vi "Speed of VIight FPGA_v4.vi"() -> ()   [LabVIEW 2026]
uses:
  <vilib>/rvi/Emulation/niFpgaGetClockAttributes.vi
  <vilib>/rvi/Emulation/niFpgaSctlEmulationGetInTimedLoop.vi
  <vilib>/rvi/Emulation/niFpgaEmulationReportErrorSimple.vi
  <instrlib>/_niInstr/Basic Elements/v1/FPGA/Private/Count Up U16.vi
  <vilib>/rvi/eio/common/nirviEmuTemplateMethod_errors.vi
  <vilib>/rvi/Emulation/niFpgaCriticalErrorInLSC.vi
  <vilib>/rvi/Emulation/niFpgaProcessEmulError.vi
  <vilib>/eio/EIONode/EIONode.xnode
  <instrlib>/_niInstr/Basic Elements/v1/FPGA/niInstr Basic Elements v1 FPGA.lvlib
panel:
  out "Play Sound 2":bool
  in  "Frequency Array":fxp<+,32,0>[](array[numeric])=[1.100008375942707e-05, 1.165410503745079e-05, 1.3081356883049011e-05, 1.3859011232852936e-05, 1.7461366951465607e-05, 1.8499791622161865e-05, 2.1999934688210487e-05, 2.330821007490158e-05, 2.6162713766098022e-05, 2.7718255296349525e-05]
  in  "Tone 1 Length":u32=15000
  out "Bonus On?":bool
  in  "Tone Length":u32=40000
  in  "Audio Loop Stop":bool
  in  "reset":bool
  out "sine out":i16
  in  "Count(uSec)":u32=10
  out "Play Sound":bool
  out "Idle Loop":i32
  in  "Period":u16=100
  in  "Idle Pattern":u16[](array[numeric])=[0, 0, 0, 0, 0, 0, 0, 0, 0, 0, 0, 0, 0, 0, 0, 0, 0, 0, 0, 0, 0, 0, 0, 0, 0, 0, 0, 0, 0, 0, 0, 0, 0, 0, 0, 0, 0, 0, 0, 0, 0, 0, 0, 0, 0]
  out "Main Loop Complete":bool
  out "Player 2 Output 5":bool[](array[boolean])
  out "Player 1 Output 5":bool[](array[boolean])
  out "Initial 6 Random Numbers":u8[](array[numeric])
  out "Player 2 Bonus":u8
  out "Player 1 Bonus":u8
  in  "Max Bonus":u8=5
  in  "Bonus Threshold":u64=3000
  out "Intial Random Arrays":u8[](array[numeric])
  out "Player2 Input":bool[](array[boolean])
  out "Player1 Input":bool[](array[boolean])
  out "Player 2 Output 4":bool[](array[boolean])
  out "Player 2 Output 3":bool[](array[boolean])
  out "Player 2 Output 2":bool[](array[boolean])
  out "Player 2 Output 1":bool[](array[boolean])
  out "Player 1 Output 4":bool[](array[boolean])
  out "Player 1 Output 3":bool[](array[boolean])
  out "Player 1 Output 2":bool[](array[boolean])
  out "Player 2 Score":u32
  out "Player 2 Timer":u64
  out "Player 1 Score":u32
  out "Player 1 Timer":u64
  out "Main Loop":i32
  out "Closing Loop":i32
  out "Element to change 2":i32
  out "Element to change":i32
  out "Measured Main Loop Ticks":u32
  in  "Main Loop Timer":u32=1 caption="Main Loop Timer (uSec)"
  out "Player2 Output Number":u32
  out "Player1 Output Number":u32
  out "Initialized Array 2":bool[](array[boolean])
  out "Initialized Array 1":bool[](array[boolean])
  out "Random Number":u8
  in  "Random Number Max":u8=20
  out "Current State":i16
  out "Blue2":bool
  out "Green3":bool
  out "Green2":bool
  out "Blue1":bool
  out "Green1":bool
  out "Player 1 Output":bool[](array[boolean])
  in  "Game Length (s)":u32=45
  in  "Stop Closing Loop":bool
  in  "Stop Main Loop":bool
  in  "Stop Idle":bool
  in  "Global Stop":bool
  # "100kHz"
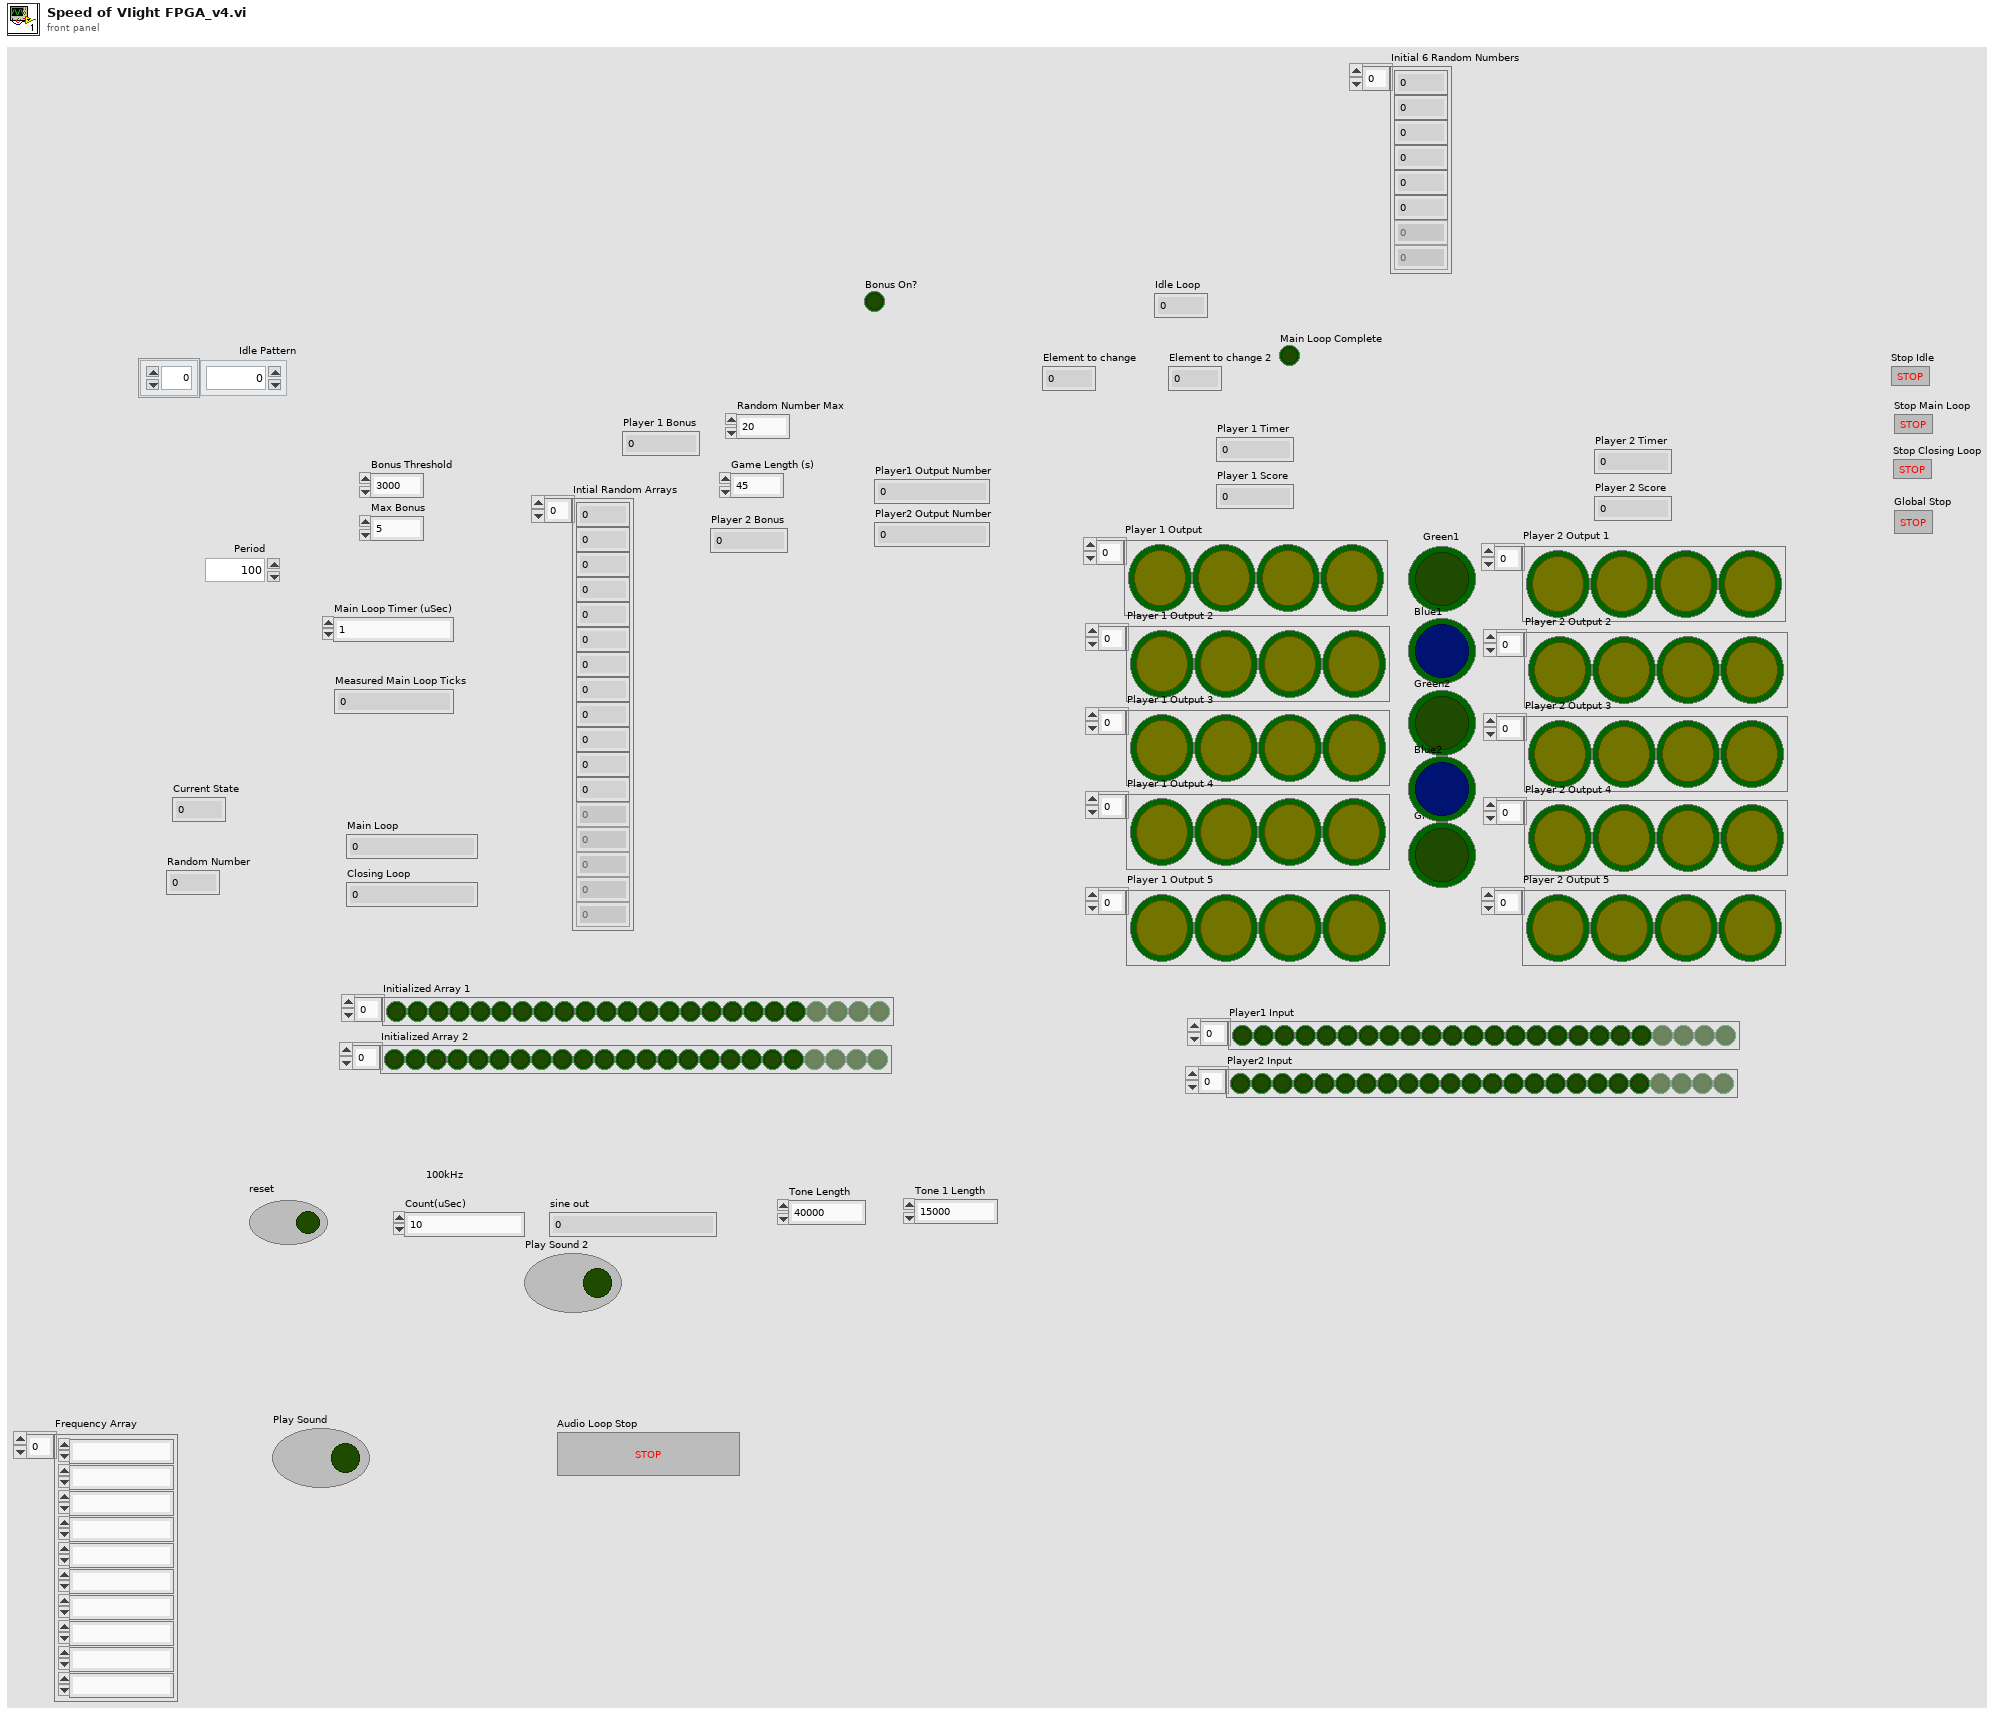
[diagram p1: front panel]
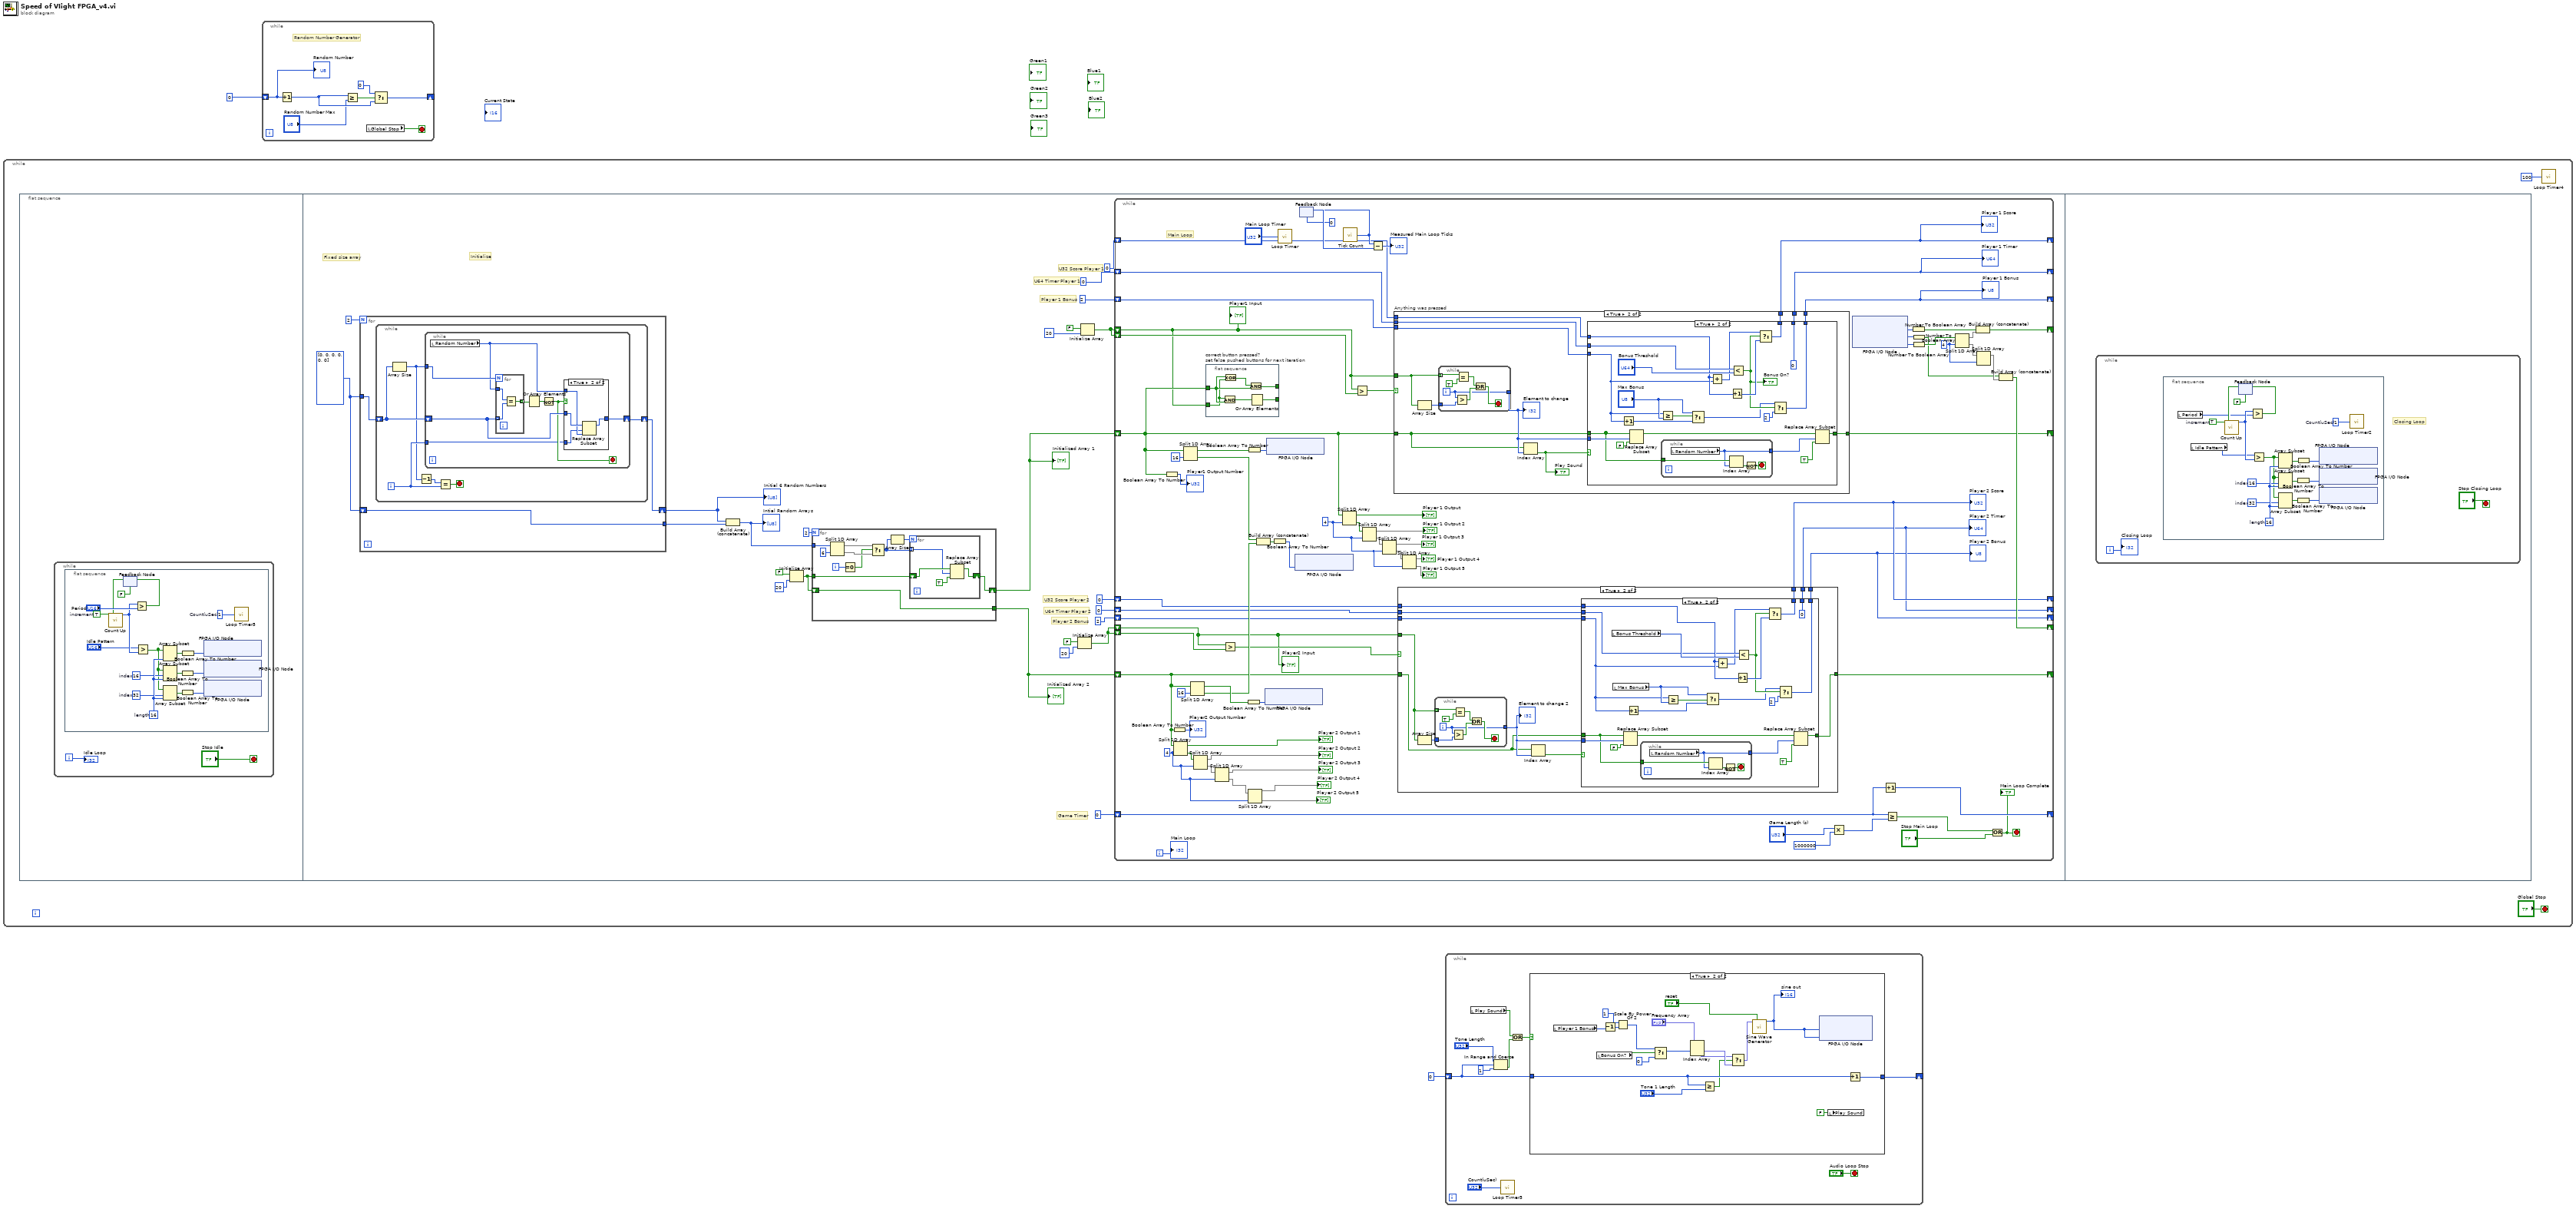
[diagram p0: block diagram]
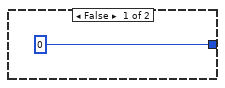
[diagram p2: hidden frame]
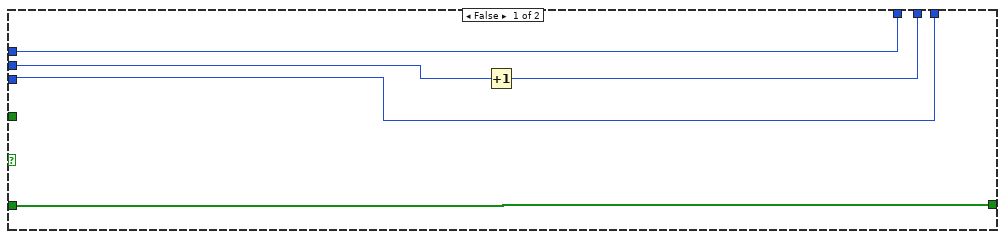
[diagram p4: hidden frame]
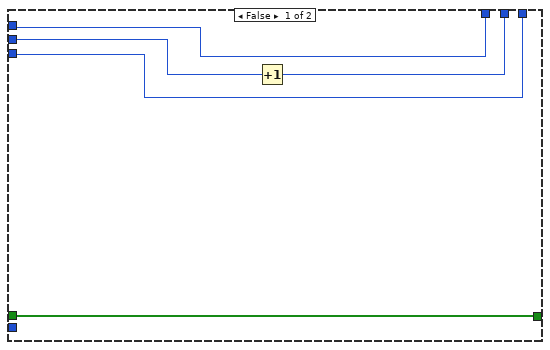
[diagram p5: hidden frame]
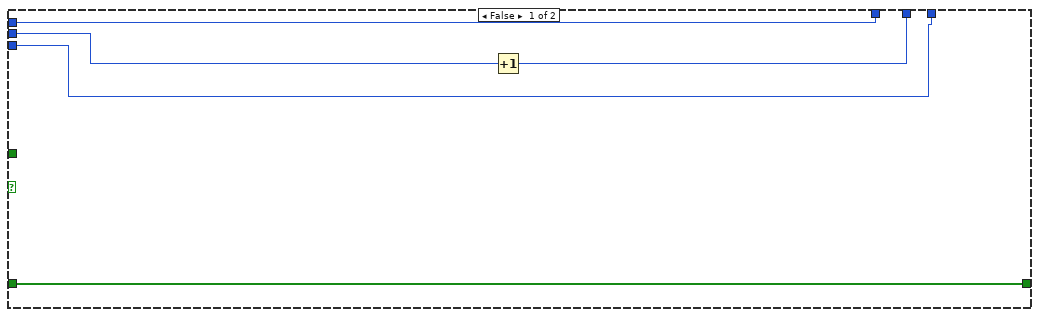
[diagram p6: hidden frame]
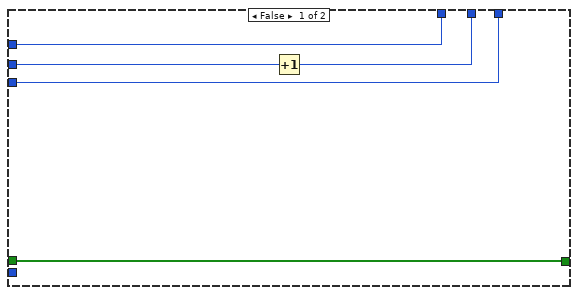
[diagram p7: hidden frame]
diagram:
  n1 = while {
    stop <- "Global Stop" stop-if-true
    n2 = flat-sequence {
      frame #0 {
        n3 = while {
          i -> [w5]
          stop <- "Stop Idle" stop-if-true
          n4 = flat-sequence {
            frame #0 {
              w11 = 32  # index
              w12 = 16  # index
              w13 = 16  # length
              w20 = u16 1  # Count(uSec)
              w23 = TRUE  # increment
              n5 = feedback #1(FALSE) -> (w19:bool)
              n6 = call-poly <instrlib>:"Count Up.vi"("increment"=w23, "reset"=w19) -> ("count out"=w18:u16)  [unwired: 13 in]
              n7 = Greater?(x=w18, y="Period") -> (0:w21:bool)
              n8 = feedback-in #1(w21) -> ()
              n9 = Greater?(x="Idle Pattern", y=w18) -> (0:w9:bool[])
              n10 = Array Subset(array=w9, length=w13) -> (w7:bool[])  [unwired: 1 in]
              n11 = Array Subset(array=w9, index=w12, length=w13) -> (w8:bool[])
              n12 = Array Subset(array=w9, index=w11, length=w13) -> (w10:bool[])
              n13 = Boolean Array To Number(Boolean array=w8) -> (number=w15:u16)
              n14 = Boolean Array To Number(Boolean array=w10) -> (number=w14:u16)
              n15 = Boolean Array To Number(Boolean array=w7) -> (number=w16:u16)
              n16 = xnode "FPGA I/O Node"("Bank-01/DO15:0"=w16) -> ()  [unwired: 1 in, 1 out]
              n17 = xnode "FPGA I/O Node"("Bank-02/DO15:0"=w15) -> ()  [unwired: 1 in, 1 out]
              n18 = xnode "FPGA I/O Node"("Bank-03/DO15:0"=w14) -> ()  [unwired: 1 in, 1 out]
              n19 = call "Loop Timer5"("Count(uSec)"=w20) -> ()  [unwired: 1 out]
            }
          }
          "Idle Loop" <- w5
        }
      }
      frame #1 {
        w30 = u8[] [0, 0, 0, 0, 0, 0] ("Initial Random Numbers")
        # "Player 2 Bonus"
        # "Player 1 Bonus"
        # "Initialize"
        # "Fixed size array"
        # "Game Timer"
        # "U32 Score Player 2"
        # "U32 Score Player 1"
        # "U64 Timer Player 2"
        # "U64 Timer Player 1"
        n20 = for {
          N: 2 -> [_]
          tunnel: w30 -> [w66]
          shift-right: [w65] -> w29
          shift-left: w30 -> [w64]
          tunnel: [w64] -> w28
          n21 = while {
            shift-right: [w69] -> w65
            shift-left: w66 -> [w70]
            i -> [w72]
            stop <- w71 stop-if-true
            n22 = Array Size(array=w70) -> (size(s)=w67:i32)
            n23 = Decrement(x=w67) -> (x-1=w68:i32)
            n24 = while {
              tunnel: w72 -> [w74]
              shift-right: [w75] -> w69
              shift-left: w70 -> [w77]
              tunnel: w67 -> [w80]
              stop <- w76 stop-if-true
              n25 = local read "Random Number"() -> (w73:u8)
              n26 = for {
                N: w80 -> [_]
                tunnel: w77 -> [w87] mode=indexing
                tunnel: w73 -> [w88]
                tunnel: [w86] -> w79 mode=indexing
                n27 = Equal?(x=w88, y=w87) -> (x = y?=w86:bool)
              }
              n28 = Or Array Elements(Boolean array=w79) -> (logical OR=w78:bool)
              n29 = Not(x=w78) -> (.not. x?=w76:bool)
              n30 = case shown="True" w76 {
                tunnel: w77 -> [w81 w85]
                tunnel: [w81 w84] -> w75
                tunnel: w73 -> [_ w83]
                tunnel: w74 -> [_ w82]
                frame False {
                }
                frame True {
                  n31 = Replace Array Subset(array=w85, new element=w83, index=w82) -> (w84:u8[])
                }
              }
            }
            n32 = Equal?(x=w68, y=w72) -> (x = y?=w71:bool)
          }
        }
        "Initial 6 Random Numbers" <- w29
        n33 = Build Array (concatenate)(w29, w28) -> (w27:u8[])
        "Intial Random Arrays" <- w27
        n34 = Initialize Array(FALSE ("Boolean"), 20 ("dimension size")) -> (w31:bool[])
        n35 = for {
          N: 2 -> [_]
          tunnel: w31 -> [w58]
          tunnel: w27 -> [w56]
          shift-right: [w59] -> w26
          shift-left: w31 -> [w49]
          tunnel: [w49] -> w25
          i -> [w52]
          n36 = Split 1D Array(array=w56, index=6) -> (first subarray=w53:u8[], second subarray=w54:u8[])
          n37 = Equal To 0?(x=w52) -> (x = 0?=w51:bool)
          n38 = Select(t=w53, s=w51, f=w54) -> (s? t:f=w50:u8[])
          n39 = Array Size(array=w50) -> (size(s)=w57:i32)
          n40 = for {
            N: w57 -> [_]
            tunnel: w50 -> [w60] mode=indexing
            shift-right: [w63] -> w59
            shift-left: w58 -> [w62]
            n41 = Replace Array Subset(array=w62, new element=TRUE ("new element/subarray"), index=w60) -> (w63:bool[])
          }
        }
        "Initialized Array 1" <- w26
        "Initialized Array 2" <- w25
        n42 = Initialize Array(FALSE ("Boolean"), 20 ("dimension size")) -> (w32:bool[])
        n43 = Initialize Array(FALSE ("Boolean"), 20 ("dimension size")) -> (w35:bool[])
        n44 = while {
          shift-right: [w110] -> _
          shift-left: u64 0 -> [w113]
          shift-right: [w104] -> _
          shift-left: u64 0 -> [w108]
          shift-right: [w111] -> _
          shift-left: u32 0 -> [w112]
          shift-right: [w105] -> _
          shift-left: u32 0 -> [w106]
          shift-right: [w164] -> _
          shift-left: u32 0 -> [w165]
          shift-right: [w134] -> _
          shift-left: w26 -> [w91]
          shift-right: [w131] -> _
          shift-left: w25 -> [w125]
          shift-right: [w139] -> _
          shift-left: w35 -> [w89]
          shift-right: [w138] -> _
          shift-left: w32 -> [w114]
          shift-left: w35 -> [w137]
          shift-left: w32 -> [w133]
          shift-right: [w109] -> _
          shift-left: u8 2 -> [w90]
          shift-right: [w103] -> _
          shift-left: u8 2 -> [w107]
          i -> [w127]
          stop <- w92 stop-if-true
          w93 = 4 ("index")
          w100 = 4 ("index")
          w145 = 4 ("index")
          # "Main Loop"
          n45 = Boolean Array To Number(Boolean array=w91) -> (number=→"Player1 Output Number":u32)
          n46 = Boolean Array To Number(Boolean array=w125) -> (number=→"Player2 Output Number":u32)
          n47 = Split 1D Array(array=w125, index=w100) -> (first subarray=→"Player 2 Output 1":bool[], second subarray=w123:bool[])
          n48 = Split 1D Array(array=w91, index=16) -> (first subarray=w135:bool[], second subarray=w155:bool[])
          n49 = Split 1D Array(array=w125, index=16) -> (first subarray=w158:bool[], second subarray=w154:bool[])
          n50 = Split 1D Array(array=w123, index=w100) -> (first subarray=→"Player 2 Output 2":bool[], second subarray=w121:bool[])
          n51 = flat-sequence "correct button pressed?\nset false pushed buttons for next iteration" {
            tunnel: [w171] -> _
            tunnel: w91 -> [w169]
            tunnel: w89 -> [w168]
            tunnel: [w167] -> _
            frame #0 {
              n52 = And(x=w168, y=w169) -> (x .and. y?=w170:bool[])
              n53 = Exclusive Or(1:w168, 2:w169) -> (0:w172:bool[])
              n54 = And(x=w172, y=w169) -> (x .and. y?=w171:bool[])
              n55 = Or Array Elements(Boolean array=w170) -> (logical OR=w167:bool)
            }
          }
          n56 = Split 1D Array(array=w121, index=w100) -> (first subarray=→"Player 2 Output 3":bool[], second subarray=w98:bool[])
          n57 = Greater?(x=w114, y=w133) -> (0:w132:bool)
          n58 = Boolean Array To Number(Boolean array=w158) -> (number=w157:u32)
          n59 = Boolean Array To Number(Boolean array=w135) -> (number=w160:u32)
          n60 = Split 1D Array(array=w98, index=w100) -> (first subarray=→"Player 2 Output 4":bool[], second subarray=→"Player 2 Output 5":bool[])
          n61 = Build Array (concatenate)(w155, w154) -> (w153:bool[])
          n62 = xnode "FPGA I/O Node"("Bank-02/DO15:0"=w157) -> ()  [unwired: 1 in, 1 out]
          n63 = xnode "FPGA I/O Node"("Bank-01/DO15:0"=w160) -> ()  [unwired: 1 in, 1 out]
          n64 = Boolean Array To Number(Boolean array=w153) -> (number=w152:u32)
          n65 = call "Loop Timer"("Count(uSec)"="Main Loop Timer") -> ()  [unwired: 1 out]
          n66 = xnode "FPGA I/O Node"("Bank-03/DO15:0"=w152) -> ()  [unwired: 1 in, 1 out]
          n67 = feedback #2(u32 0) -> (w142:u32)
          n68 = Split 1D Array(array=w91, index=w93) -> (first subarray=→"Player 1 Output":bool[], second subarray=w119:bool[])
          n69 = call "Tick Count"() -> ("Tick Count(Ticks)"=w141:u32)
          n70 = feedback-in #2(w141) -> ()
          n71 = Greater?(x=w89, y=w137) -> (0:w136:bool)
          n72 = Split 1D Array(array=w119, index=w93) -> (first subarray=→"Player 1 Output 2":bool[], second subarray=w118:bool[])
          n73 = Subtract(x=w141, y=w142) -> (x-y=→"Measured Main Loop Ticks":u32)
          n74 = Split 1D Array(array=w118, index=w93) -> (first subarray=→"Player 1 Output 3":bool[], second subarray=w96:bool[])
          n75 = case "Anything was pressed" shown="True" w136 {
            tunnel: [w232 w244] -> w134
            tunnel: w89 -> [_ w242]
            tunnel: w91 -> [w232 w240]
            tunnel: w113 -> [w230 w236]
            tunnel: [w229 w238] -> w110
            tunnel: w112 -> [w231 w237]
            tunnel: [w231 w239] -> w111
            tunnel: w90 -> [w228 w235]
            tunnel: [w228 w234] -> w109
            frame False {
              n76 = Increment(x=w230) -> (x+1=w229:u64)
            }
            frame True {
              n77 = Array Size(array=w242) -> (size(s)=w241:i32)
              n78 = while {
                tunnel: w242 -> [w282] mode=indexing
                tunnel: w241 -> [w278]
                tunnel: [w276] -> w243
                i -> [w276]
                stop <- w279 stop-if-true
                n79 = Greater?(x=w276, y=w278) -> (0:w277:bool)
                n80 = Equal?(x=w282, y=TRUE ("element")) -> (x = y?=w280:bool)
                n81 = Or(x=w280, y=w277) -> (x .or. y?=w279:bool)
              }
              "Element to change" <- w243
              n82 = Index Array(array=w240, index=w243) -> (element=w233:bool)
              "Play Sound" <- w233
              n83 = case shown="True" w233 {
                tunnel: w243 -> [_ w271]
                tunnel: [w249 w267] -> w244
                tunnel: w240 -> [w249 w265]
                tunnel: w237 -> [w248 w252]
                tunnel: w236 -> [w247 w263]
                tunnel: [w248 w261] -> w239
                tunnel: [w246 u64 0] -> w238
                tunnel: w235 -> [w245 w251]
                tunnel: [w245 w258] -> w234
                frame False {
                  n84 = Increment(x=w247) -> (x+1=w246:u64)
                }
                frame True {
                  n85 = Increment(x=w251) -> (x+1=w254:u8)
                  n86 = Replace Array Subset(array=w265, new element=FALSE ("new element/subarray"), index=w271) -> (w269:bool[])
                  n87 = Greater Or Equal?(x=w251, y="Max Bonus") -> (x >= y?=w256:bool)
                  n88 = while {
                    tunnel: [w272] -> w266
                    tunnel: w265 -> [w275]
                    stop <- w273 stop-if-true
                    n89 = local read "Random Number"() -> (w272:u8)
                    n90 = Index Array(array=w275, index=w272) -> (element=w274:bool)
                    n91 = Not(x=w274) -> (.not. x?=w273:bool)
                  }
                  n92 = Select(t="Max Bonus", s=w256, f=w254) -> (s? t:f=w253:u8)
                  n93 = Add(x=w252, y=w251) -> (x+y=w250:u32)
                  n94 = Increment(x=w252) -> (x+1=w262:u32)
                  n95 = Less?(x=w263, y="Bonus Threshold") -> (x < y?=w260:bool)
                  "Bonus On?" <- w260
                  n96 = Select(t=w250, s=w260, f=w262) -> (s? t:f=w261:u32)
                  n97 = Select(t=w253, s=w260, f=u8 2) -> (s? t:f=w258:u8)
                  n98 = Replace Array Subset(array=w269, new element=TRUE ("new element/subarray"), index=w266) -> (w267:bool[])
                }
              }
            }
          }
          "Player 1 Timer" <- w110
          "Player 1 Score" <- w111
          "Player 1 Bonus" <- w109
          n99 = case shown="True" w132 {
            tunnel: [w177 w185] -> w131
            tunnel: w114 -> [_ w187]
            tunnel: w125 -> [w177 w184]
            tunnel: w108 -> [w175 w182]
            tunnel: w107 -> [w173 w181]
            tunnel: w106 -> [w176 w183]
            tunnel: [w176 w179] -> w105
            tunnel: [w174 w180] -> w104
            tunnel: [w173 w178] -> w103
            frame False {
              n100 = Increment(x=w175) -> (x+1=w174:u64)
            }
            frame True {
              n101 = Array Size(array=w187) -> (size(s)=w186:i32)
              n102 = while {
                tunnel: w187 -> [w227] mode=indexing
                tunnel: w186 -> [w223]
                tunnel: [w221] -> w189
                i -> [w221]
                stop <- w224 stop-if-true
                n103 = Greater?(x=w221, y=w223) -> (0:w222:bool)
                n104 = Equal?(x=w227, y=TRUE ("element")) -> (x = y?=w225:bool)
                n105 = Or(x=w225, y=w222) -> (x .or. y?=w224:bool)
              }
              "Element to change 2" <- w189
              n106 = Index Array(array=w184, index=w189) -> (element=w188:bool)
              n107 = case shown="True" w188 {
                tunnel: w189 -> [_ w216]
                tunnel: [w194 w212] -> w185
                tunnel: w184 -> [w194 w210]
                tunnel: w183 -> [w190 w202]
                tunnel: w182 -> [w193 w197]
                tunnel: w181 -> [w191 w195]
                tunnel: [w192 u64 0] -> w180
                tunnel: [w191 w200] -> w178
                tunnel: [w190 w199] -> w179
                frame False {
                  n108 = Increment(x=w193) -> (x+1=w192:u64)
                }
                frame True {
                  n109 = local read "Bonus Threshold"() -> (w204:u64)
                  n110 = local read "Max Bonus"() -> (w203:u8)
                  n111 = Replace Array Subset(array=w210, new element=FALSE ("new element/subarray"), index=w216) -> (w214:bool[])
                  n112 = Increment(x=w195) -> (x+1=w198:u8)
                  n113 = while {
                    tunnel: [w217] -> w211
                    tunnel: w210 -> [w220]
                    stop <- w218 stop-if-true
                    n114 = local read "Random Number"() -> (w217:u8)
                    n115 = Index Array(array=w220, index=w217) -> (element=w219:bool)
                    n116 = Not(x=w219) -> (.not. x?=w218:bool)
                  }
                  n117 = Greater Or Equal?(x=w195, y=w203) -> (x >= y?=w206:bool)
                  n118 = Select(t=w203, s=w206, f=w198) -> (s? t:f=w205:u8)
                  n119 = Add(x=w202, y=w195) -> (x+y=w196:u32)
                  n120 = Increment(x=w202) -> (x+1=w209:u32)
                  n121 = Less?(x=w197, y=w204) -> (x < y?=w208:bool)
                  n122 = Select(t=w196, s=w208, f=w209) -> (s? t:f=w199:u32)
                  n123 = Select(t=w205, s=w208, f=u8 2) -> (s? t:f=w200:u8)
                  n124 = Replace Array Subset(array=w214, new element=TRUE ("new element/subarray"), index=w211) -> (w212:bool[])
                }
              }
            }
          }
          "Player 2 Timer" <- w104
          "Player 2 Score" <- w105
          "Player 2 Bonus" <- w103
          n125 = Split 1D Array(array=w96, index=w93) -> (first subarray=→"Player 1 Output 4":bool[], second subarray=→"Player 1 Output 5":bool[])
          n126 = Multiply(x="Game Length (s)", y=u32 1000000) -> (x*y=w128:u32)
          n127 = xnode "FPGA I/O Node"() -> ("Bank-01/DI15:0"=w151:u16, "Bank-02/DI15:0"=w150:u16, "Bank-03/DI15:0"=w149:u16)  [unwired: 3 in, 3 out]
          n128 = Increment(x=w165) -> (x+1=w164:u32)
          n129 = Greater Or Equal?(x=w165, y=w128) -> (x >= y?=w163:bool)
          n130 = Number To Boolean Array(number=w151) -> (Boolean array=w147:bool[])
          n131 = Number To Boolean Array(number=w150) -> (Boolean array=w101:bool[])
          n132 = Number To Boolean Array(number=w149) -> (Boolean array=w102:bool[])
          n133 = Split 1D Array(array=w102, index=w145) -> (first subarray=w146:bool[], second subarray=w144:bool[])
          n134 = Build Array (concatenate)(w147, w146) -> (w139:bool[])
          n135 = Split 1D Array(array=w144, index=w145) -> (first subarray=w143:bool[])  [unwired: 1 out]
          n136 = Or(x=w163, y="Stop Main Loop") -> (x .or. y?=w92:bool)
          "Main Loop Complete" <- w92
          n137 = Build Array (concatenate)(w101, w143) -> (w138:bool[])
          "Main Loop" <- w127
          "Player1 Input" <- w89
          "Player2 Input" <- w114
        }
      }
      frame #2 {
        n138 = while {
          i -> [w283]
          stop <- "Stop Closing Loop" stop-if-true
          # "Closing Loop"
          n139 = flat-sequence {
            frame #0 {
              w291 = 32  # index
              w292 = 16  # index
              w293 = 16  # length
              w299 = u16 1  # Count(uSec)
              w302 = TRUE  # increment
              n140 = local read "Period"() -> (w285:u16)
              n141 = local read "Idle Pattern"() -> (w286:u16[])
              n142 = feedback #3(FALSE) -> (w298:bool)
              n143 = call-poly <instrlib>:"Count Up.vi"("increment"=w302, "reset"=w298) -> ("count out"=w297:u16)  [unwired: 13 in]
              n144 = Greater?(x=w297, y=w285) -> (0:w300:bool)
              n145 = feedback-in #3(w300) -> ()
              n146 = Greater?(x=w286, y=w297) -> (0:w289:bool[])
              n147 = Array Subset(array=w289, length=w293) -> (w287:bool[])  [unwired: 1 in]
              n148 = Array Subset(array=w289, index=w292, length=w293) -> (w288:bool[])
              n149 = Array Subset(array=w289, index=w291, length=w293) -> (w290:bool[])
              n150 = Boolean Array To Number(Boolean array=w288) -> (number=w295:u16)
              n151 = Boolean Array To Number(Boolean array=w290) -> (number=w294:u16)
              n152 = Boolean Array To Number(Boolean array=w287) -> (number=w296:u16)
              n153 = xnode "FPGA I/O Node"("Bank-01/DO15:0"=w296) -> ()  [unwired: 1 in, 1 out]
              n154 = xnode "FPGA I/O Node"("Bank-02/DO15:0"=w295) -> ()  [unwired: 1 in, 1 out]
              n155 = xnode "FPGA I/O Node"("Bank-03/DO15:0"=w294) -> ()  [unwired: 1 in, 1 out]
              n156 = call "Loop Timer2"("Count(uSec)"=w299) -> ()  [unwired: 1 out]
            }
          }
          "Closing Loop" <- w283
        }
      }
    }
    n157 = call "Loop Timer4"("Count(mSec)"=u32 100 ("millisecond multiple")) -> ()  [unwired: 1 out]
  }
  n158 = while {
    shift-right: [w307] -> _
    shift-left: u8 0 -> [w309]
    stop <- w303 stop-if-true
    # "Random Number Generator"
    n159 = Increment(x=w309) -> (x+1=w306:u8)
    n160 = Greater Or Equal?(x=w306, y="Random Number Max") -> (x >= y?=w305:bool)
    n161 = local read "Global Stop"() -> (w303:bool)
    n162 = Select(t=u8 0, s=w305, f=w306) -> (s? t:f=w307:u8)
    "Random Number" <- w309
  }
  n163 = while {
    shift-right: [w316] -> _
    shift-left: u32 0 -> [w312]
    stop <- "Audio Loop Stop" stop-if-true
    n164 = local read "Play Sound"() -> (w314:bool)
    n165 = In Range and Coerce(upper limit="Tone Length", x=w312, lower limit=u32 1) -> (In Range?=w310:bool)  [unwired: 1 out]
    n166 = call "Loop Timer3"("Count(uSec)"="Count(uSec)") -> ()  [unwired: 1 out]
    n167 = Or(x=w314, y=w310) -> (x .or. y?=w315:bool)
    n168 = case shown="True" w315 {
      tunnel: w312 -> [_ w328]
      tunnel: [i16 0 w335] -> w316
      frame False {
      }
      frame True {
        n169 = local read "Player 1 Bonus"() -> (w333:u8)
        n170 = local read "Bonus On?"() -> (w334:bool)
        n171 = Decrement(x=w333) -> (x-1=w322:u8)
        n172 = Scale By Power Of 2(n=i16 1, x=w322) -> (x*2^n=w320:u8)
        n173 = Select(t=w320, s=w334, f=u8 0) -> (s? t:f=w331:u8)
        n174 = Index Array(array="Frequency Array", index #1=w331) -> (element #1=w330:fxp<+,32,0>, element #2=w329:fxp<+,32,0>)  [unwired: 1 in]
        n175 = Greater Or Equal?(x=w328, y="Tone 1 Length") -> (x >= y?=w327:bool)
        n176 = Select(t=w329, s=w327, f=w330) -> (s? t:f=w326:fxp<+,32,0>)
        n177 = call "Sine Wave Generator"("frequency (periods/tick)"=w326, "reset"="reset") -> ("sine out"=w336:i16)  [unwired: 13 in]
        "sine out" <- w336
        n178 = xnode "FPGA I/O Node"("SteroOut/AO0"=w336, "SteroOut/AO1"=w336) -> ()  [unwired: 2 in, 2 out]
        n179 = local write "Play Sound"(FALSE ("Play Sound")) -> ()
        n180 = Increment(x=w328) -> (x+1=w335:u32)
      }
    }
  }
